vi "采样频率.vi"(11 "采样频率 f/Hz":string(combo)="5") -> ()   [LabVIEW 2016]
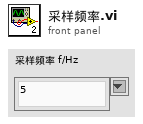
[diagram p1: front panel]
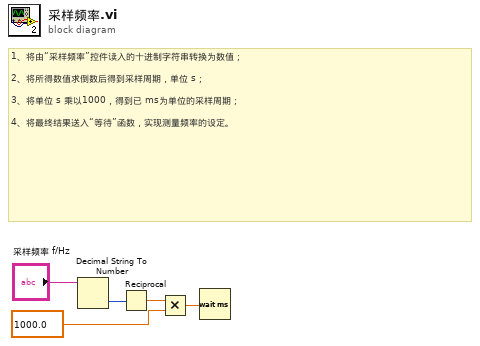
[diagram p0: block diagram]
diagram:
  # "1、将由“采样频率”控件读入的十进制字符串转换为数值；\n\n2、将所得数值求倒数后得到采样周期，单位 s；\n\n3、将单位 s 乘以1000，得到已 ms为单位的采样周期；\n\n4、将最终结果送入“等待”函数，实现测量频率的设定。"
  n1 = Decimal String To Number(string="采样频率 f/Hz") -> (number=w3:i32)  [unwired: 2 in, 1 out]
  n2 = Reciprocal(x=w3) -> (1/x=w4:dbl)
  n3 = Multiply(x=w4, y=1000.0) -> (x*y=w2:dbl)
  n4 = Wait (ms)(milliseconds to wait=w2) -> ()  [unwired: 1 out]
